vi "Receive.vi"(6 "Timeout":T2={"mode"=enum."Relative", "deadline (ms)"=30000}, 8 "error in (no error)":errorcluster, 9 "request id":u32, 10 "session in":refnum<class "Session.lvclass">, 11 "NI_SFTP.lvlib:statvfs_openssh.com.lvclass":refnum<class "statvfs_openssh.com.lvclass">) -> (0 "error out":errorcluster, 1 "statistics":T1 {"f_flag" format="%x"; "f_fsid" format="%x"}, 2 "session out":refnum<class "Session.lvclass">, 3 "NI_SFTP.lvlib:statvfs_openssh.com.lvclass 2":refnum<class "statvfs_openssh.com.lvclass">)   [LabVIEW 2020, in "NI_SFTP.lvlib" / "statvfs_openssh.com.lvclass"]
uses:
  <vilib>/net/SFTP/API/Support/Command/statvfs_openssh.com/statvfs_openssh.com.lvclass
  <vilib>/net/SFTP/Session/Session.lvclass
  <vilib>/Utility/Deadline/Deadline.ctl
  <vilib>/Utility/Deadline/Mode.ctl
  <vilib>/net/SFTP/API/Support/statvfs info.ctl
  <vilib>/net/SFTP/API/Support/Command/SSH_FXP_EXTENDED/SSH_FXP_EXTENDED.lvclass
  <vilib>/net/SFTP/NI_SFTP.lvlib
  <vilib>/Utility/Deadline/NI_Deadline.lvlib
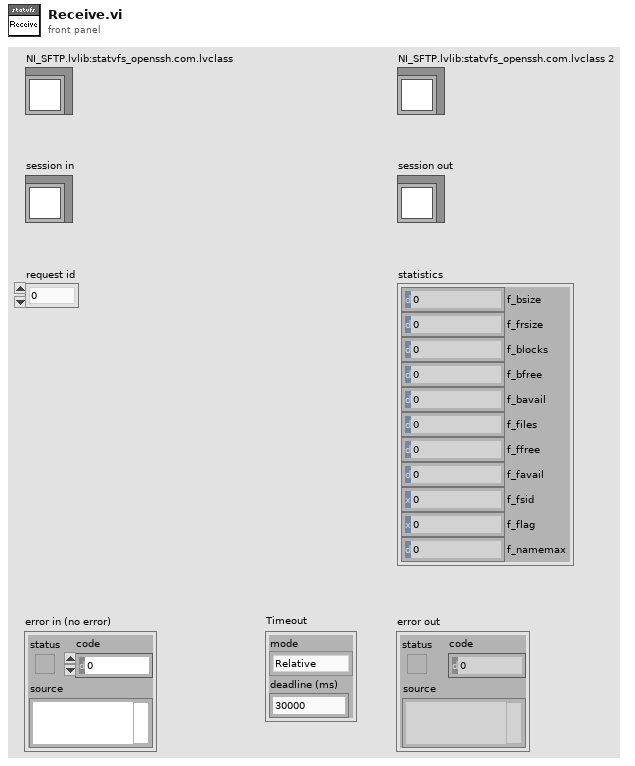
[diagram p1: front panel]
types:
  T1 = typedef "NI_SFTP.lvlib/statvfs info.ctl" = cluster{"f_bsize":u64, "f_frsize":u64, "f_blocks":u64, "f_bfree":u64, "f_bavail":u64, "f_files":u64, "f_ffree":u64, "f_favail":u64, "f_fsid":u64, "f_flag":u64, "f_namemax":u64}
  T2 = typedef "NI_Deadline.lvlib/Deadline.ctl" = cluster{"mode":T3, "deadline (ms)":u32}
  T3 = typedef "NI_Deadline.lvlib/Mode.ctl" = enum16{"Relative", "Use deadline", "Wait forever", "Nonblocking", "N/A"}
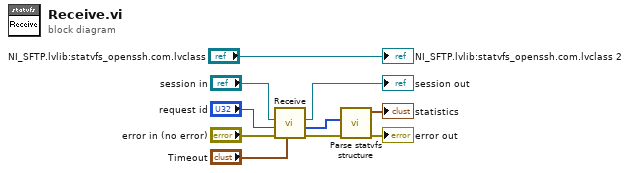
[diagram p0: block diagram]
diagram:
  n1 = call <vilib>:"Receive.vi"("deadline"="Timeout", "error in (no error)"="error in (no error)", "request id"="request id", "session in"="session in") -> ("error out"=w6:errorcluster, "payload"=w2:u8[], "session out"=→"session out":refnum<class "Session.lvclass">)  [unwired: 4 in, 1 out]
  n2 = call <vilib>:"Parse statvfs structure.vi"("error in (no error)"=w6, "payload"=w2) -> ("error out"=→"error out":errorcluster, "statvfs"=→"statistics":T1)  [unwired: 8 in]
  "NI_SFTP.lvlib:statvfs_openssh.com.lvclass 2" <- "NI_SFTP.lvlib:statvfs_openssh.com.lvclass"
